vi "load_recipes.vi"(8 "error in (no error)":errorcluster, 11 "recipe":T2) -> (0 "error out":errorcluster, 2 "transition []":string, 3 "recipe []":T1[](array[typedef]))   [LabVIEW 2015, in "example_01.lvlib"]
uses:
  example_01.lvlib
  _controls/recipes.ctl
  lv-recipe-machine/public/_controls/recipe_step.ctl
  _controls/steps_actions.ctl
  lv-recipe-machine/lv-recipe-machine.lvlib
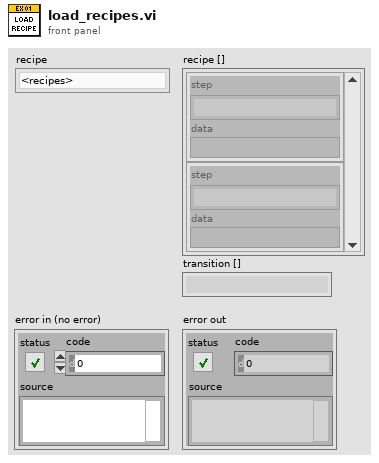
[diagram p1: front panel]
types:
  T1 = typedef "lv-recipe-machine.lvlib/recipe_step.ctl" = cluster{"step":string, "data":variant}
  T2 = typedef "example_01.lvlib/recipes.ctl" = enum16{"<recipes>", "wait_random", "random_wait", "count", "comparison", "<null>"}
  T3 = typedef "example_01.lvlib/steps_actions.ctl" = enum16{"<steps_actions>", "manual_random", "manual_comparison", "manual_wait", "auto_random", "auto_wait", "criteria_initialize", "criteria_count", "criteria_comparison", "transition_simple", "transition_count", "transition_comparison", "<null>"}
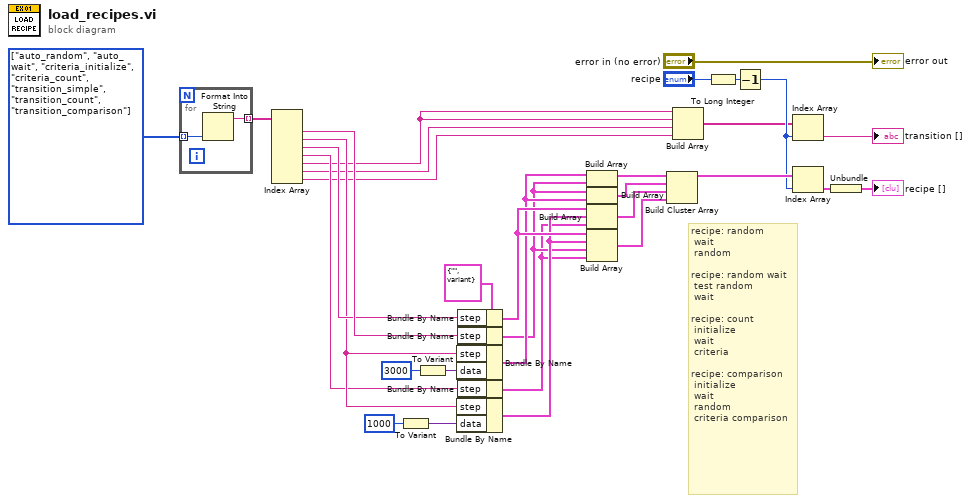
[diagram p0: block diagram]
diagram:
  w17 = T3[] [enum."auto_random", enum."auto_wait", enum."criteria_initialize", enum."criteria_count", enum."transition_simple", enum."transition_count", enum."transition_comparison"] items=["<steps_actions>", "manual_random", "manual_comparison", "manual_wait", "auto_random", "auto_wait", "criteria_initialize", "criteria_count", "criteria_comparison", "transition_simple", "transition_count", "transition_comparison", "<null>"]
  w10 = T1 {"step"="", "data"=variant} ("lv-recipe-machine.lvlib:recipe_step")
  # "recipe: random\n wait\n random \n\nrecipe: random wait\n test random\n wait\n\nrecipe: count\n initialize\n wait\n criteria\n\nrecipe: comparison\n initialize\n wait\n random\n criteria comparison"
  n1 = for {
    tunnel: w17 -> [w34] mode=indexing
    tunnel: [w33] -> w16 mode=indexing
    n2 = Format Into String(w34) -> (resulting string=w33:string)  [unwired: 3 in, 1 out]
  }
  n3 = Index Array(array=w16) -> (element #1=w15:string, element #2=w13:string, element #3=w14:string, element #4=w12:string, element #5=w3:string, element #6=w2:string, element #7=w1:string)  [unwired: 7 in]
  n4 = To Variant(anything=1000) -> (Variant=w20:variant)
  n5 = To Variant(anything=3000) -> (Variant=w31:variant)
  n6 = Bundle By Name(cluster=w10, "step"=w13, "data"=w31) -> (w6:T1)
  n7 = Bundle By Name(cluster=w10, "step"=w13, "data"=w20) -> (w7:T1)
  n8 = Bundle By Name(cluster=w10, "step"=w14) -> (w9:T1)
  n9 = Bundle By Name(cluster=w10, "step"=w15) -> (w5:T1)
  n10 = Bundle By Name(cluster=w10, "step"=w12) -> (w4:T1)
  n11 = Build Array(w6, w5) -> (w22:T1[])
  n12 = Build Array(w5, w6) -> (w21:T1[])
  n13 = Build Array(w9, w7, w4) -> (w18:T1[])
  n14 = Build Array(w9, w7, w5, w4) -> (w8:T1[])
  n15 = Build Cluster Array(w22, w21, w18, w8) -> (w30:cluster{T1[]}[])
  n16 = Build Array(w3, w3, w2, w1) -> (w11:string[])
  n17 = To Long Integer(number="recipe") -> (32bit integer=w27:i32)
  n18 = Decrement(x=w27) -> (x-1=w24:i32)
  n19 = Index Array(array=w11, index=w24) -> (element=→"transition []":string)
  n20 = Index Array(array=w30, index=w24) -> (element=w26:cluster{T1[]})
  n21 = Unbundle(w26) -> (→"recipe []":T1[])
  "error out" <- "error in (no error)"
